vi "Stop Type set.vi"(5 "Stop way":enum16{"OUTOFF", "ALARM", "BEEPER"}(ring), 6 "ON/OFF(T:ON F:OFF)":bool, 7 "Channel  (1: CH1)":u16(ring)=1 items=["CH1"=1, "CH2"=2, "CH3"=3, "CH4"=4], 8 "error in (no error)":errorcluster, 11 "VISA resource in":refnum<visa-resource-name>) -> (0 "error out":errorcluster, 3 "VISA resource name out":refnum<visa-resource-name>)   [LabVIEW 2020, in "GPP.lvlib"]
uses:
  GPP.lvlib
  Function/VISA_COMMON.ctl
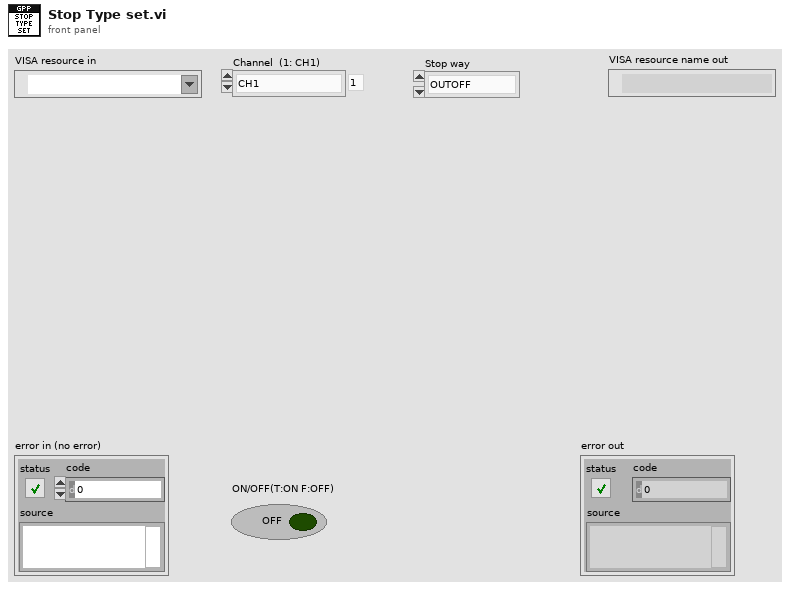
[diagram p1: front panel]
types:
  T1 = typedef "GPP.lvlib/VISA_COMMON.ctl" = enum16{"Initial", "Write CMD", "Read Result", "Read History", "Close"}
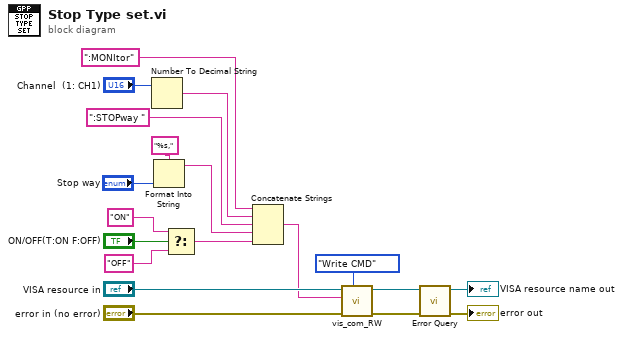
[diagram p0: block diagram]
diagram:
  n1 = Number To Decimal String(number="Channel  (1: CH1)") -> (decimal integer string=w10:string)  [unwired: 1 in]
  n2 = Format Into String(format string="%s,", "Stop way") -> (resulting string=w3:string)  [unwired: 2 in, 1 out]
  n3 = Select(t="ON", s="ON/OFF(T:ON F:OFF)", f="OFF") -> (s? t:f=w2:string)
  n4 = Concatenate Strings(":MONItor", w10, ":STOPway ", w3, w2) -> (w5:string)
  n5 = call "vis_com_RW.vi"("Funciton"=VISA_COMMON."Write CMD", "error in (no error)"="error in (no error)", "CMD String"=w5, "VISA resource in"="VISA resource in") -> ("error out"=w18:errorcluster, "VISA resource out"=w19:refnum<visa-resource-name>)  [unwired: 5 in, 1 out]
  n6 = call "Error Query.vi"("error in (no error)"=w18, "VISA resource name"=w19) -> ("error out"=→"error out":errorcluster, "VISA resource name out"=→"VISA resource name out":refnum<visa-resource-name>)  [unwired: 6 in, 2 out]
